vi "Create List.vi"(8 "error in (no error)":errorcluster, 9 "List type":i32(ring) items=["Number", "Bullet"], 10 "list elements":string[](array[string]), 11 "ooWriter in":refnum<class "ooCalc.lvclass">) -> (0 "error out":errorcluster, 2 "List":refnum<k24>, 3 "ooWriter out":refnum<class "ooCalc.lvclass">)   [LabVIEW 2009, in "ooCalc.lvclass"]
uses:
  ooCalc.lvclass
  C:/Projets/LAVAG/OpenOfficeRGT/AODL/DLLs/AODL.dll
  ooCalc.lvclass/ooCalc.ctl
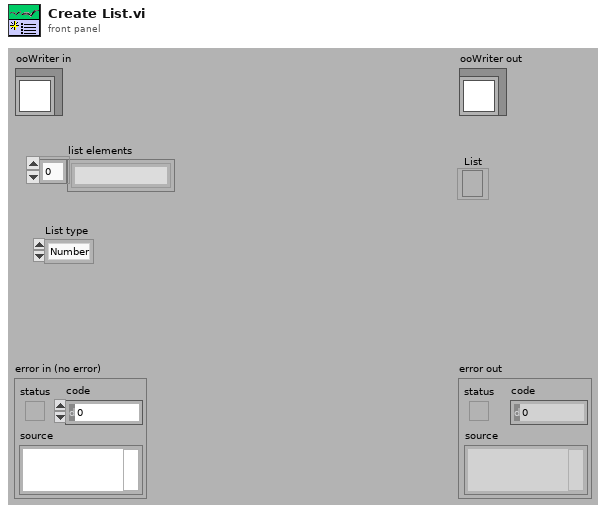
[diagram p1: front panel]
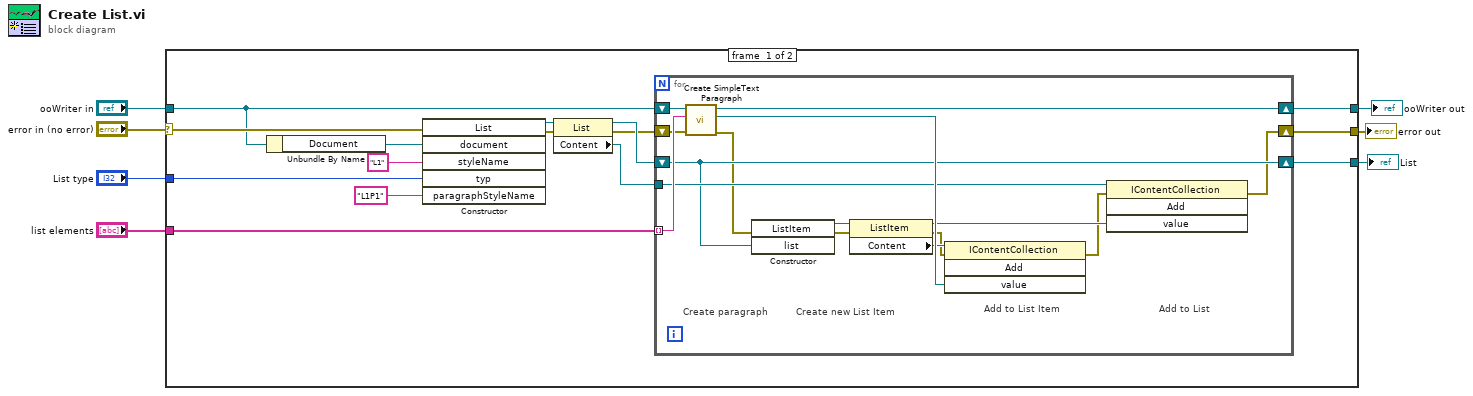
[diagram p0: block diagram]
diagram:
  n1 = case shown="No Error" "error in (no error)" {
    selector: "error in (no error)" -> [w13 w39]
    tunnel: [w11 w39] -> w6
    tunnel: [w9 w38] -> w4
    tunnel: "ooWriter in" -> [w10 w38]
    tunnel: "List type" -> [w14 _]
    tunnel: "list elements" -> [w12 _]
    tunnel: [w8 _] -> w1
    frame #0 {
      n2 = Unbundle By Name(w10) -> ("Document"=w22:refnum<k24>)
      n3 = constructor class="List"(error in=w13, "document"=w22, "styleName"="L1", "typ"=w14, "paragraphStyleName"="L1P1") -> (reference out=w17:refnum<k24>, error out=w16:errorcluster)  [unwired: 2 in, 5 out]
      n4 = property class="List"(reference=w17, error in=w16) -> (reference out=w18:refnum<k24>, error out=w15:errorcluster, "Content"=w19:refnum<k24>)
      n5 = for {
        tunnel: w12 -> [w36] mode=indexing
        shift-right: [w35] -> w9
        shift-left: w10 -> [w37]
        tunnel: w19 -> [w31]
        shift-right: [w28] -> w8
        shift-left: w18 -> [w28]
        shift-right: [w26] -> w11
        shift-left: w15 -> [w23]
        # "Add to List"
        # "Create new List Item"
        # "Add to List Item"
        # "Create paragraph"
        n6 = call-dynamic "Create SimpleText Paragraph.vi"("error in (no error)"=w23, "simpleText"=w36, "ooWriter in"=w37) -> ("error out"=w24:errorcluster, "SimpleTextParagraph"=w34:refnum<k24>, "ooWriter out"=w35:refnum<class "ooCalc.lvclass">)  [unwired: 6 in]
        n7 = constructor class="ListItem"(error in=w24, "list"=w28) -> (reference out=w33:refnum<k24>, error out=w27:errorcluster)  [unwired: 2 in, 2 out]
        n8 = property class="ListItem"(reference=w33, error in=w27) -> (reference out=w30:refnum<k24>, error out=w25:errorcluster, "Content"=w32:refnum<k24>)
        n9 = invoke class="IContentCollection" method="Add"(reference=w32, error in=w25, "value"=w34) -> (error out=w29:errorcluster)  [unwired: 1 in, 3 out]
        n10 = invoke class="IContentCollection" method="Add"(reference=w31, error in=w29, "value"=w30) -> (error out=w26:errorcluster)  [unwired: 1 in, 3 out]
      }
    }
    frame #1 {
    }
  }
  "error out" <- w6
  "ooWriter out" <- w4
  "List" <- w1
